vi "Read Excel Sheet.vi"(8 "error in (no error)":errorcluster, 11 "Path":path) -> (0 "error out":errorcluster, 3 "Array":string[][](array[string]))   [LabVIEW 2017, in "Localization.lvlib" / "Excel Support.lvlib"]
doc: "<B>Description:</B> Reads the first Sheet of an Excel File as strings.\n\n<B>Date:</B> 11/2022\n<B>Author:</B> Luke Jarocki, Choose Movement Consulting"
uses:
  Excel Support.lvlib
  Microsoft.Office.Interop.Excel
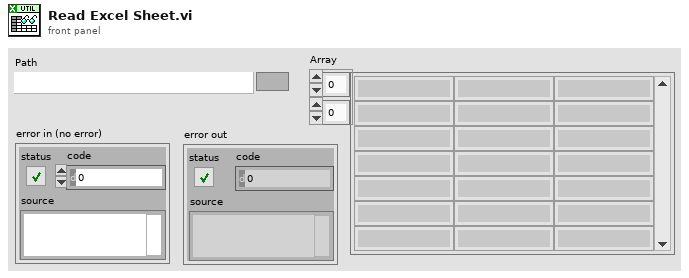
[diagram p1: front panel]
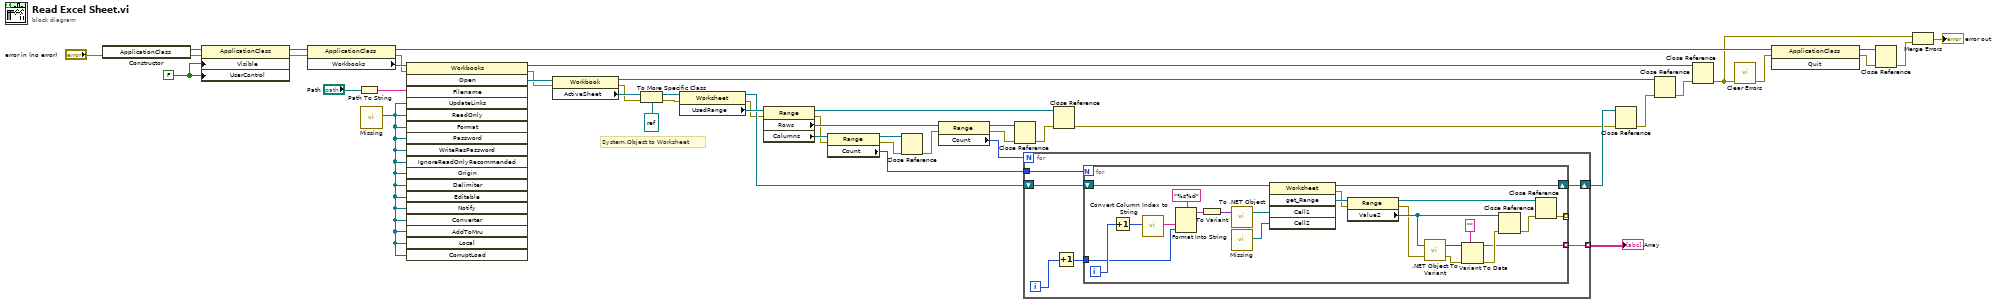
[diagram p0: block diagram]
diagram:
  w44 = FALSE ("Visible (F)")
  # "System.Object to Worksheet"
  n1 = constructor class="ApplicationClass"(error in="error in (no error)") -> (reference out=w17:refnum<k24>, error out=w18:errorcluster)  [unwired: 2 in, 1 out]
  n2 = property class="ApplicationClass"(reference=w17, error in=w18, "Visible"=w44, "UserControl"=w44) -> (reference out=w16:refnum<k24>, error out=w13:errorcluster)
  n3 = property class="ApplicationClass"(reference=w16, error in=w13) -> (reference out=w3:refnum<k24>, error out=w12:errorcluster, "Workbooks"=w47:refnum<k24>)
  n4 = Path To String(path="Path") -> (string=w46:string)
  n5 = call "Missing.vi"() -> ("Missing"=w25:refnum<k24>)  [unwired: 11 in]
  n6 = invoke class="Workbooks" method="Open"(reference=w47, error in=w12, "Filename"=w46, "UpdateLinks"=w25, "ReadOnly"=w25, "Format"=w25, "Password"=w25, "WriteResPassword"=w25, "IgnoreReadOnlyRecommended"=w25, "Origin"=w25, "Delimiter"=w25, "Editable"=w25, "Notify"=w25, "Converter"=w25, "AddToMru"=w25, "Local"=w25, "CorruptLoad"=w25) -> (reference out=w43:refnum<k24>, error out=w11:errorcluster, "Open"=w45:refnum<k24>)  [unwired: 1 in, 15 out]
  n7 = property class="Workbook"(reference=w45, error in=w11) -> (reference out=w41:refnum<k24>, error out=w10:errorcluster, "ActiveSheet"=w38:refnum<k24>)
  n8 = To More Specific Class(target class=refnum<k24> refnum ("reference out"), reference=w38, error in=w10) -> (specific class reference=w37:refnum<k24>, error out=w9:errorcluster)
  n9 = property class="Worksheet"(reference=w37, error in=w9) -> (reference out=w26:refnum<k24>, error out=w8:errorcluster, "UsedRange"=w36:refnum<k24>)
  n10 = property class="Range"(reference=w36, error in=w8) -> (reference out=w28:refnum<k24>, error out=w7:errorcluster, "Rows"=w35:refnum<k24>, "Columns"=w34:refnum<k24>)
  n11 = property class="Range"(reference=w34, error in=w7) -> (reference out=w31:refnum<k24>, error out=w22:errorcluster, "Count"=w29:i32)
  n12 = Close Reference(reference=w31, error in (no error)=w22) -> (error out=w21:errorcluster)
  n13 = property class="Range"(reference=w35, error in=w21) -> (reference out=w33:refnum<k24>, error out=w32:errorcluster, "Count"=w30:i32)
  n14 = Close Reference(reference=w33, error in (no error)=w32) -> (error out=w27:errorcluster)
  n15 = for {
    N: w30 -> [_]
    tunnel: w29 -> [w53]
    shift-right: [w50] -> w24
    shift-left: w26 -> [w52]
    tunnel: [w49] -> w23 mode=indexing
    i -> [w51]
    n16 = Increment(x=w51) -> (x+1=w48:i32)
    n17 = for {
      N: w53 -> [_]
      tunnel: w48 -> [w73]
      shift-right: [w68] -> w50
      shift-left: w52 -> [w76]
      tunnel: [w59] -> w49 mode=indexing
      tunnel: [w55] -> _ mode=indexing
      i -> [w75]
      n18 = Increment(x=w75) -> (x+1=w56:i32)
      n19 = call "Convert Column Index to String.vi"("Column Index (1)"=w56) -> ("Column Letter"=w58:string)  [unwired: 10 in]
      n20 = Format Into String(format string="%s%d", w58, w73) -> (resulting string=w71:string)  [unwired: 2 in, 1 out]
      n21 = To Variant(anything=w71) -> (Variant=w72:variant)
      n22 = call <vilib>:"To .NET Object.vi"("anything"=w72) -> (".NET object"=w70:refnum<k24>)  [unwired: 1 in, 1 out]
      n23 = call "Missing.vi"() -> ("Missing"=w69:refnum<k24>)  [unwired: 11 in]
      n24 = invoke class="Worksheet" method="get_Range"(reference=w76, "Cell1"=w70, "Cell2"=w69) -> (reference out=w68:refnum<k24>, error out=w54:errorcluster, "get_Range"=w67:refnum<k24>)  [unwired: 2 in, 2 out]
      n25 = property class="Range"(reference=w67, error in=w54) -> (reference out=w63:refnum<k24>, error out=w57:errorcluster, "Value2"=w60:refnum<k24>)
      n26 = call <vilib>:".NET Object To Variant.vi"("error in (no error)"=w57, ".NET object"=w60) -> ("error out"=w65:errorcluster, "variant"=w66:variant)
      n27 = Variant To Data(error in=w65, type="", Variant=w66) -> (data=w59:string, error out=w62:errorcluster)
      n28 = Close Reference(reference=w60, error in (no error)=w62) -> (error out=w61:errorcluster)
      n29 = Close Reference(reference=w63, error in (no error)=w61) -> (error out=w55:errorcluster)
    }
  }
  "Array" <- w23
  n30 = Close Reference(reference=w28, error in (no error)=w27) -> (error out=w20:errorcluster)
  n31 = Close Reference(reference=w24, error in (no error)=w20) -> (error out=w39:errorcluster)
  n32 = Close Reference(reference=w41, error in (no error)=w39) -> (error out=w42:errorcluster)
  n33 = Close Reference(reference=w43, error in (no error)=w42) -> (error out=w2:errorcluster)
  n34 = call <vilib>:"Clear Errors.vi"("error in (no error)"=w2) -> ("error out"=w1:errorcluster)  [unwired: 5 in, 1 out]
  n35 = invoke class="ApplicationClass" method="Quit"(reference=w3, error in=w1) -> (reference out=w4:refnum<k24>, error out=w5:errorcluster)  [unwired: 1 in, 1 out]
  n36 = Close Reference(reference=w4, error in (no error)=w5) -> (error out=w6:errorcluster)
  n37 = Merge Errors(w2, w6) -> (→"error out":errorcluster)
